vi "Measurement UI.vi"() -> ()   [LabVIEW 2024, in "NIScopeTimeDomain.lvlib"]
uses:
  NIScopeTimeDomain.lvlib
panel:
  out "Voltage Waveform Duty Cycle (%)":dbl
  out "Voltage Waveform Period (s)":dbl
  out "Voltage Frequency (Hz)":dbl
  out "Vpp Amplitude (V)":dbl
  out "Mean DC Voltage (V)":dbl
  in  "Trigger Level (V)":dbl format="%.2g"
  out "Waveform Data":dbl[](array[numeric])
  out "Voltage Waveform":waveform(dbl)(graph)
  in  "Trigger Slope":i32(ring) items=["Positive", "Negative"]
  in  "Trigger Coupling":u32(ring)=1 items=["AC"=0, "DC"=1, "HF Reject"=3, "LF Reject"=4, "AC Plus HF Reject"=1001]
  in  "Minimum Record Length (S)":dbl=10000.0
  in  "Minimum Sample Rate (S/s)":dbl=10000000.0 format="%#.2p"
  in  "Vertical Coupling":i32(ring)=1 items=["AC", "DC", "Ground"]
  in  "Vertical Offset (V)":dbl format="%.2p"
  in  "Vertical Range (V)":dbl=10.0 caption="Vertical Range" format="%.2f"
  in  "Pin Name":string(combo)
  # "Setup"
  # "Output"
  # "Input"
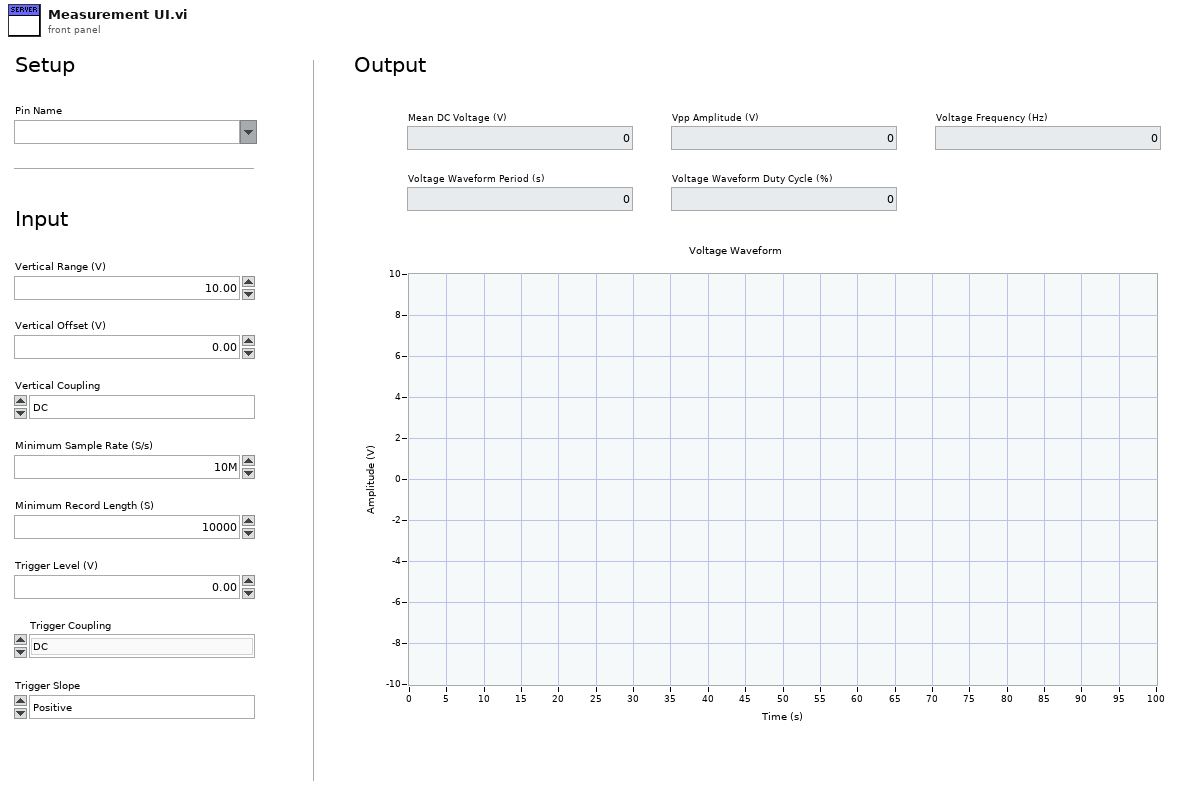
[diagram p1: front panel]
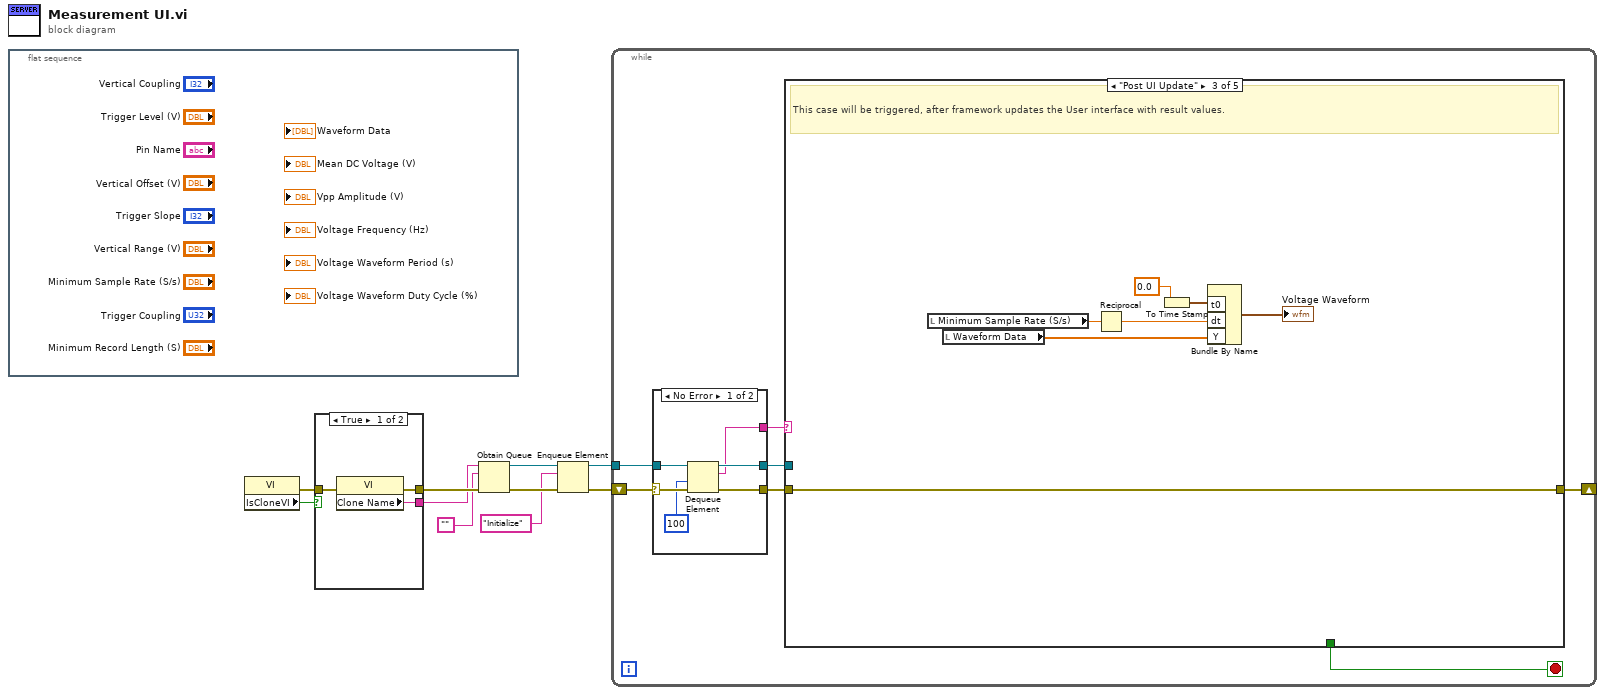
[diagram p0: block diagram]
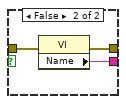
[diagram p2: hidden frame]
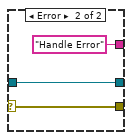
[diagram p3: hidden frame]
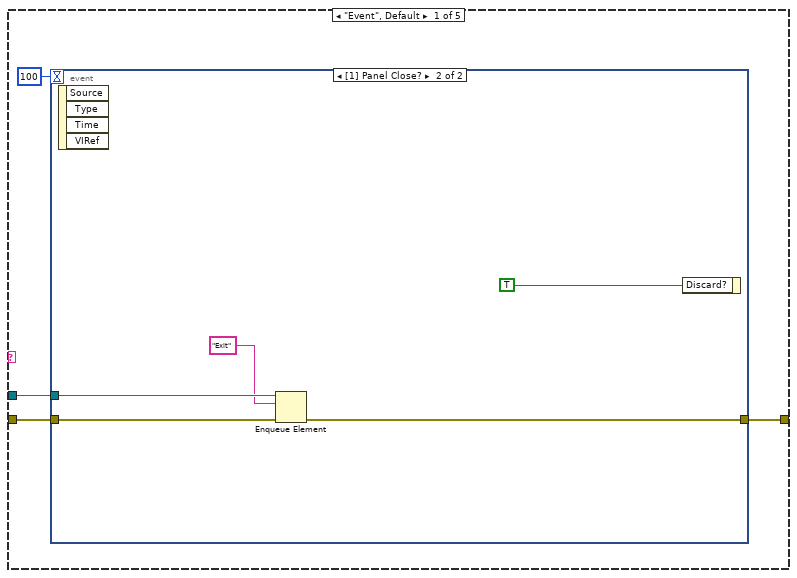
[diagram p4: hidden frame]
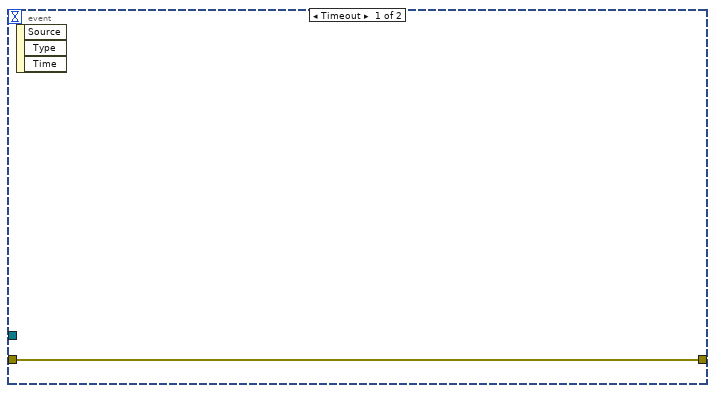
[diagram p5: hidden frame]
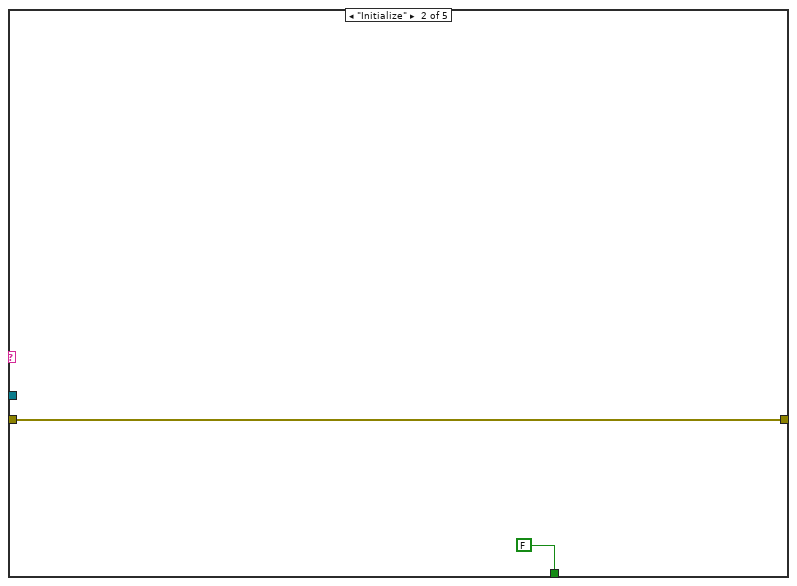
[diagram p6: hidden frame]
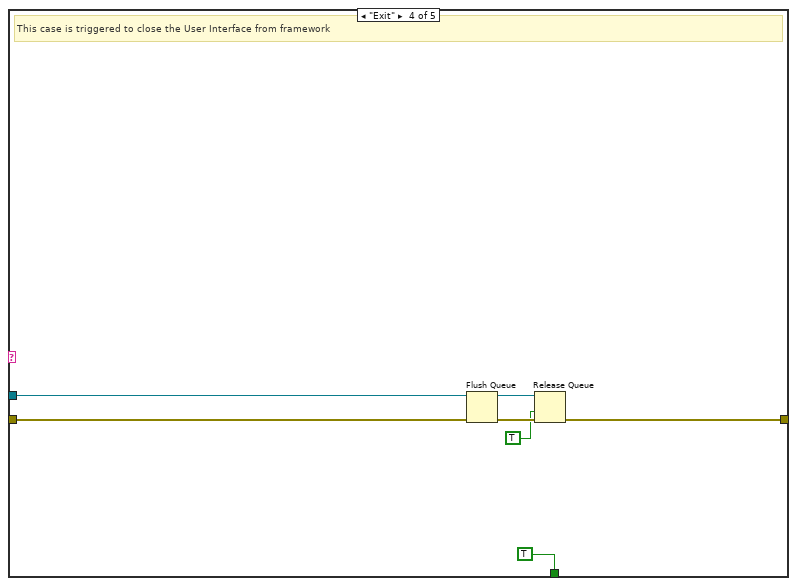
[diagram p7: hidden frame]
diagram:
  n1 = flat-sequence {
    frame #0 {
    }
  }
  n2 = property class="VI"() -> (error out=w1:errorcluster, "IsCloneVI"=w2:bool)  [unwired: 2 in, 1 out]
  n3 = case shown="True" w2 {
    tunnel: [w13 w16] -> w10
    tunnel: [w12 w15] -> w9
    tunnel: w1 -> [w11 w14]
    frame True {
      n4 = property class="VI"(error in=w11) -> (error out=w13:errorcluster, "Clone Name"=w12:string)  [unwired: 1 in, 1 out]
    }
    frame False {
      n5 = property class="VI"(error in=w14) -> (error out=w16:errorcluster, "Name"=w15:string)  [unwired: 1 in, 1 out]
    }
  }
  n6 = Obtain Queue(name (unnamed)=w9, element data type="", error in (no error)=w10) -> (queue out=w6:refnum<queue>, error out=w8:errorcluster)  [unwired: 2 in, 1 out]
  n7 = Enqueue Element(queue=w6, element="Initialize", error in (no error)=w8) -> (queue out=w5:refnum<queue>, error out=w7:errorcluster)  [unwired: 1 in, 1 out]
  n8 = while {
    shift-right: [w18] -> _
    shift-left: w7 -> [w23]
    tunnel: w5 -> [w21]
    stop <- w17 stop-if-true
    n9 = case shown="No Error" w23 {
      selector: w23 -> [w29 w32]
      tunnel: [w28 w32] -> w22
      tunnel: w21 -> [w27 w31]
      tunnel: [w26 w31] -> w20
      tunnel: [w25 "Handle Error"] -> w19
      frame No Error {
        n10 = Dequeue Element(queue=w27, timeout in ms (-1)=100, error in (no error)=w29) -> (queue out=w26:refnum<queue>, element=w25:string, error out=w28:errorcluster)  [unwired: 1 out]
      }
      frame Error {
      }
    }
    n11 = case shown="\"Post UI Update\"" w19 {
      tunnel: w22 -> [w35 w44 w51 w58 w59]
      tunnel: w20 -> [w33 _ _ w56 _]
      tunnel: [w36 w44 w51 w53 w59] -> w18
      tunnel: [_ FALSE _ TRUE _] -> w17
      frame "Event", Default {
        n12 = event shown="[1] Panel Close?" {
          selector: _ -> [_ _]
          dyn-events: _ -> [_ _]
          timeout: 100 -> [_ _]
          tunnel: [w37 w40] -> w36
          tunnel: w35 -> [w37 w41]
          tunnel: w33 -> [_ w39]
          event Timeout {
            n13 = event-data() -> ()  [unwired: 1 in, 3 out]
          }
          event Panel Close? {
            n14 = event-data() -> ()  [unwired: 1 in, 4 out]
            n15 = Enqueue Element(queue=w39, element="Exit", error in (no error)=w41) -> (error out=w40:errorcluster)  [unwired: 1 in, 2 out]
            n16 = event-data("Discard?"=TRUE) -> ()  [unwired: 1 in, 1 out]
          }
        }
      }
      frame "Initialize" {
      }
      frame "Post UI Update" {
        # "This case will be triggered, after framework updates the User interface with result values."
        n17 = local read "Minimum Sample Rate (S/s)"() -> (w50:dbl)
        n18 = local read "Waveform Data"() -> (w46:dbl[])
        n19 = Reciprocal(x=w50) -> (1/x=w47:dbl)
        n20 = To Time Stamp(1:0.0 ("t0")) -> (0:w48:timestamp)
        n21 = Bundle By Name("t0"=w48, "dt"=w47, "Y"=w46) -> (→"Voltage Waveform":waveform(dbl))  [unwired: 1 in]
      }
      frame "Exit" {
        # "This case is triggered to close the User Interface from framework"
        n22 = Flush Queue(queue=w56, error in (no error)=w58) -> (queue out=w55:refnum<queue>, error out=w54:errorcluster)  [unwired: 1 out]
        n23 = Release Queue(queue=w55, force destroy? (F)=TRUE, error in (no error)=w54) -> (error out=w53:errorcluster)  [unwired: 2 out]
      }
      frame "Handle Error" {
      }
    }
  }
